vi "Create.vi"(10 "Task Run Info":T1[](array[typedef])) -> (3 "TaskRunInfoArrayValue out":refnum<class "TaskRunInfoArrayValue.lvclass">)   [LabVIEW 2020, in "Volatus.lvlib" / "TaskRunInfoArrayValue.lvclass"]
uses:
  TaskRunInfoArrayValue.lvclass
  TaskRunInfoArrayValue.lvclass/TaskRunInfoArrayValue.ctl
  Task Hierarchy.ctl
  Volatus.lvlib
  Task State.ctl
  Task Run Info.ctl
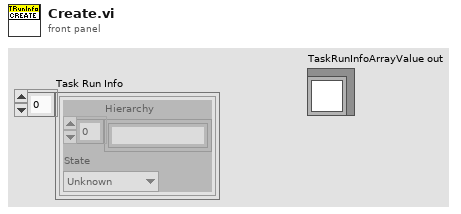
[diagram p1: front panel]
types:
  T1 = typedef "Volatus.lvlib/Task Run Info.ctl" = cluster{"Hierarchy":T2, "State":T3}
  T2 = typedef "Volatus.lvlib/Task Hierarchy.ctl" = string[]
  T3 = typedef "Volatus.lvlib/Task State.ctl" = enum16{"Unknown", "Idle", "Initializing", "Starting", "Running", "Stopping", "Stopped", "Error - Init", "Error - Start", "Error - Run", "Error - Stop"}
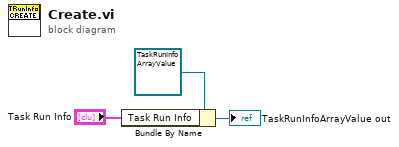
[diagram p0: block diagram]
diagram:
  n1 = Bundle By Name(cluster=refnum<class "TaskRunInfoArrayValue.lvclass"> refnum ("TaskRunInfoArrayValue in"), "Task Run Info"="Task Run Info") -> (→"TaskRunInfoArrayValue out":refnum<class "TaskRunInfoArrayValue.lvclass">)
